vi "dialog test.vi"() -> ()   [LabVIEW 2013]
panel:
  out "LabVIEW Text":string
  in  "hb":bool=TRUE
  in  "h ts":timestamp=timestamp(3523589884.3778296 s since 1904-01-01)
  in  "h num":dbl=34.0
  in  "h str":string="asdassasd"
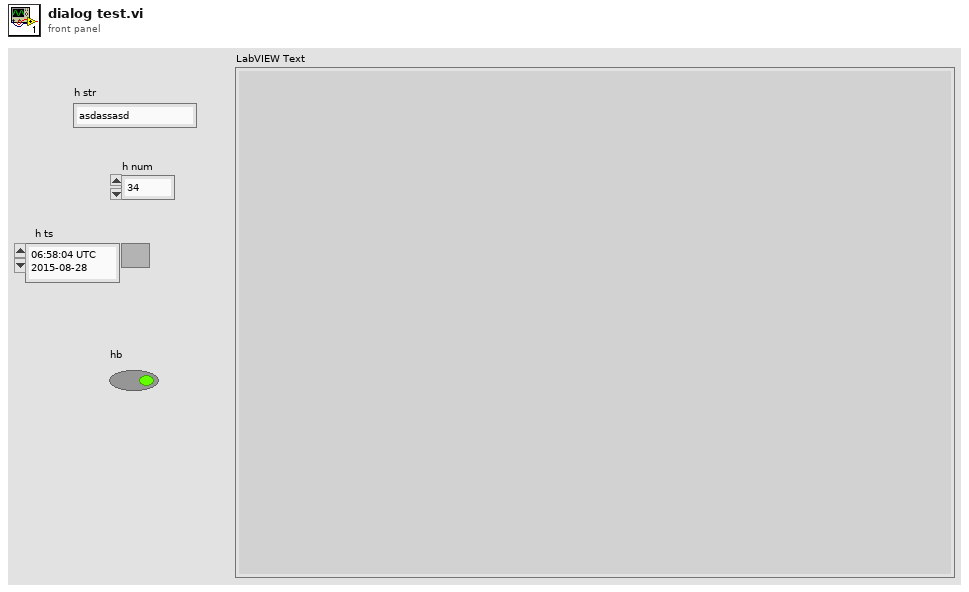
[diagram p1: front panel]
types:
  T1 = typedef "exception.lvlib/exception.ctl" = cluster{"code":i32, "context":T2, "properties":variant}
  T2 = typedef "exception.lvlib/context.ctl" = enum16{"developer", "user interface", "standard", "limited", "deterministic"}
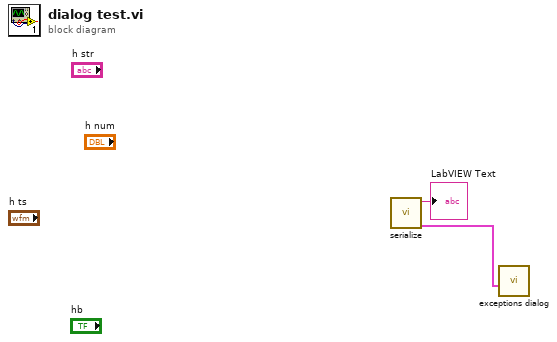
[diagram p0: block diagram]
diagram:
  n1 = call "serialize.vi"() -> ("exception out"=w2:T1, "LabVIEW Text"=→"LabVIEW Text":string)  [unwired: 10 in]
  n2 = call "exceptions dialog.vi"("exception"=w2) -> ()  [unwired: 11 in]
